vi "Parse-attribute.vi"(8 "error in (no error)":errorcluster, 10 "String in":string, 11 "TransformEnable in":refnum<class "TransformEnable.lvclass">) -> (0 "error out":errorcluster, 1 "Valid attribute?":bool, 2 "Remaining string":string, 3 "TransformEnable out":refnum<class "TransformEnable.lvclass">)   [LabVIEW 2013, in "HardwareCharacterization.lvlib" / "TransformEnable.lvclass"]
uses:
  TransformEnable.lvclass
  Attributes.ctl
  Attribute-ID.ctl
  Attribute-XML.lvclass/Attribute-XML.ctl
  ID.lvclass/ID.ctl
  Boolean/Boolean.lvclass/Boolean.ctl
  Write Attribute.vi
  Write ID-attribute.vi
  Boolean/Write Boolean.vi
  Attribute-XML.lvclass
  ID.lvclass
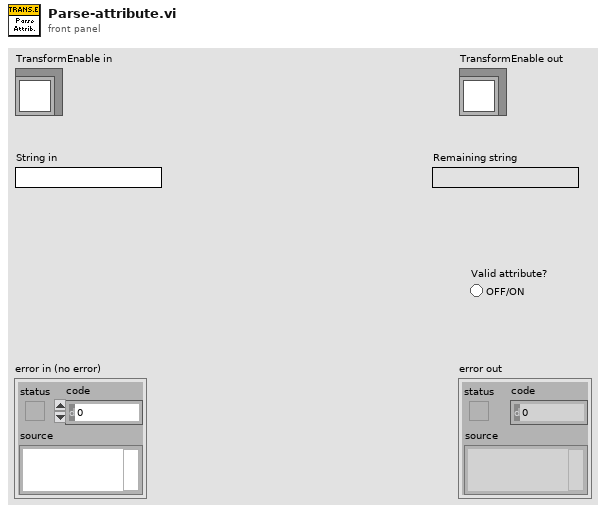
[diagram p1: front panel]
types:
  T1 = typedef "HardwareCharacterization.lvlib/ID.lvclass/Attribute-ID.ctl" = enum16{"FieldOffset", "TransformEnable", "Transform", "Units", "XYCalFactor", "EnableLaser", "JumpDelay", "MarkDelay", "PolyDelay", "LaserOnDelay", "LaserOffDelay", "JumpSpeed", "MarkSpeed", "LaserPowerDelay", "LaserEnableDelay", "LaserPower", "Offset"}
  T2 = typedef "HardwareCharacterization.lvlib/Attribute-XML.lvclass/Attributes.ctl" = enum16{"id"}
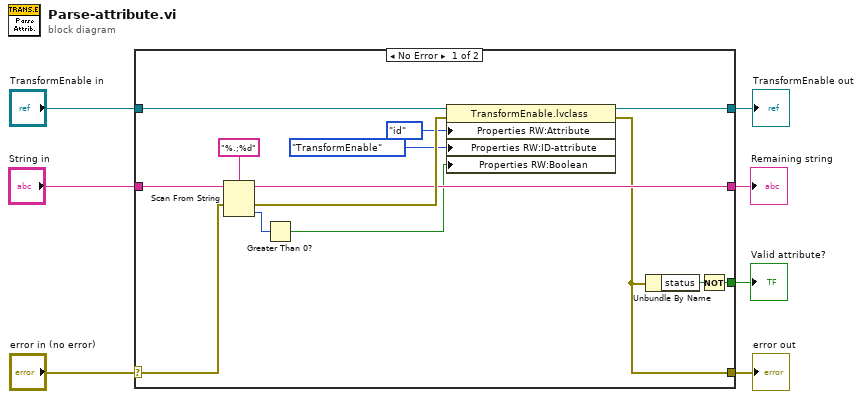
[diagram p0: block diagram]
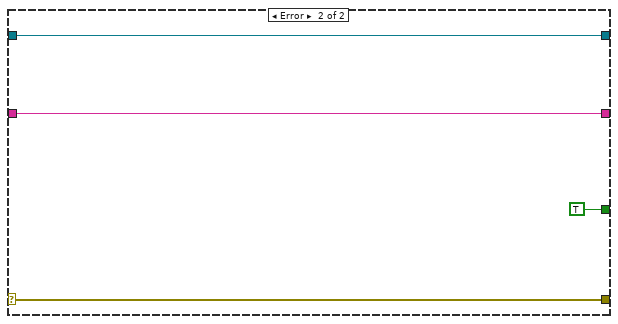
[diagram p2: hidden frame]
diagram:
  n1 = case shown="No Error" "error in (no error)" {
    selector: "error in (no error)" -> [w12 w25]
    tunnel: [w11 w25] -> w6
    tunnel: [w15 w24] -> w4
    tunnel: "TransformEnable in" -> [w16 w24]
    tunnel: "String in" -> [w14 w23]
    tunnel: [w13 w23] -> w2
    tunnel: [w10 TRUE] -> w1
    frame No Error {
      n2 = Scan From String(format string="%.;%d", input string=w14, error in=w12) -> (remaining string=w13:string, error out=w19:errorcluster, output 1=w9:i32)  [unwired: 2 in, 1 out]
      n3 = Greater Than 0?(x=w9) -> (x > 0?=w8:bool)
      n4 = property class="TransformEnable.lvclass"(reference=w16, error in=w19, "Properties RW:Attribute"=Attributes."id" ("Attribute"), "Properties RW:ID-attribute"=Attribute-ID."TransformEnable" ("ID-attribute"), "Properties RW:Boolean"=w8) -> (reference out=w15:refnum<class "TransformEnable.lvclass">, error out=w11:errorcluster)
      n5 = Unbundle By Name(w11) -> ("status"=w20:bool)
      n6 = Not(x=w20) -> (.not. x?=w10:bool)
    }
    frame Error {
    }
  }
  "error out" <- w6
  "TransformEnable out" <- w4
  "Remaining string" <- w2
  "Valid attribute?" <- w1
